vi "Math-Column Sum.vi"(1 "2D Array":dbl[][](array[numeric])) -> (0 "Column sums":dbl[](array[numeric]))   [LabVIEW 2020]
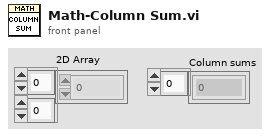
[diagram p1: front panel]
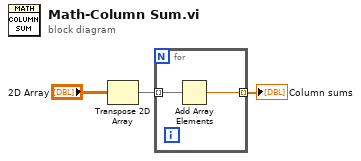
[diagram p0: block diagram]
diagram:
  n1 = Transpose 2D Array(2D array="2D Array") -> (transposed array=w2:dbl[][])
  n2 = for {
    tunnel: w2 -> [w5] mode=indexing
    tunnel: [w4] -> w1 mode=indexing
    n3 = Add Array Elements(numeric array=w5) -> (sum=w4:dbl)
  }
  "Column sums" <- w1
